vi "Find Xbee.vi"(8 "error out":errorcluster, 11 "Aircraft COM Port":refnum<visa-resource-name>) -> (0 "error out 2":errorcluster, 2 "Xbee Found":bool, 3 "Aircraft COM Port 2":refnum<visa-resource-name>)   [LabVIEW 2014]
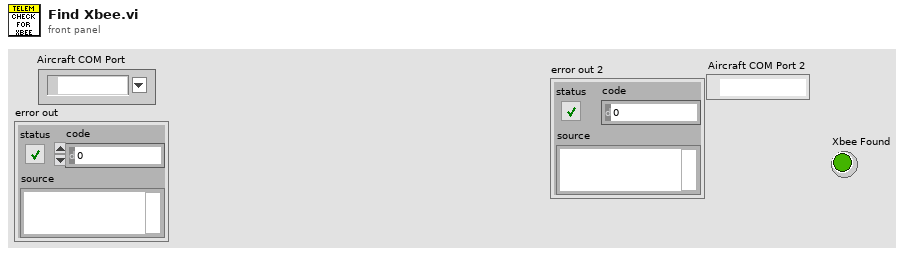
[diagram p1: front panel]
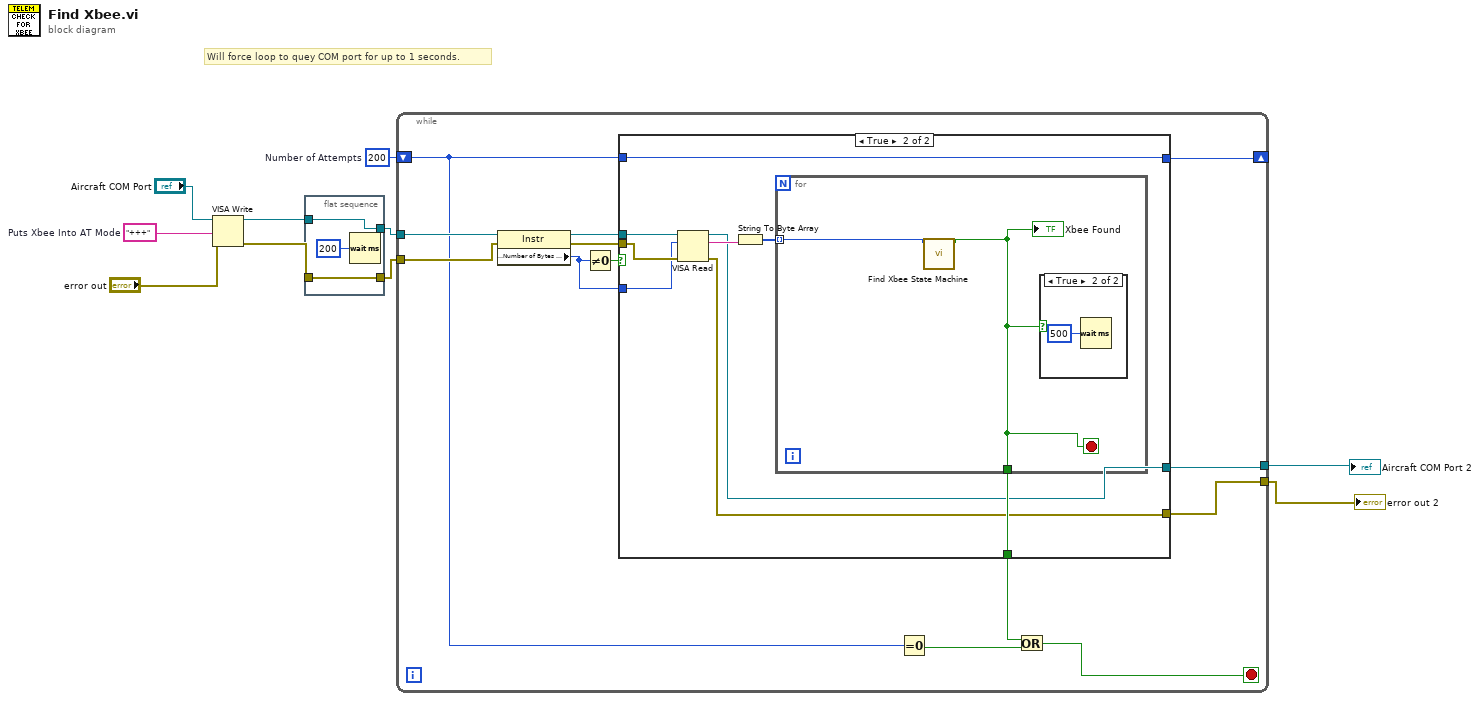
[diagram p0: block diagram]
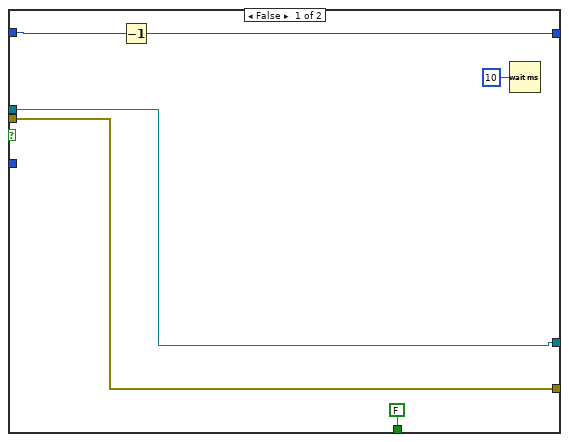
[diagram p2: hidden frame]
diagram:
  w9 = "+++"  # Puts Xbee Into AT Mode
  w10 = 200  # Number of Attempts
  # "Will force loop to quey COM port for up to 1 seconds."
  n1 = VISA Write(VISA resource name="Aircraft COM Port", write buffer=w9, error in (no error)="error out") -> (VISA resource name out=w8:refnum<visa-resource-name>, error out=w6:errorcluster)  [unwired: 1 out]
  n2 = flat-sequence {
    tunnel: w8 -> [w12]
    tunnel: [w12] -> w7
    tunnel: w6 -> [w11]
    tunnel: [w11] -> w5
    frame #0 {
      n3 = Wait (ms)(milliseconds to wait=u32 200) -> ()  [unwired: 1 out]
    }
  }
  n4 = while {
    tunnel: w7 -> [w26]
    tunnel: w5 -> [w25]
    tunnel: [w20] -> w1
    tunnel: [w19] -> w2
    shift-right: [w18] -> _
    shift-left: w10 -> [w14]
    stop <- w15 stop-if-true
    n5 = property class="Instr"(reference=w26, error in=w25) -> (reference out=w23:refnum<visa-resource-name>, error out=w22:errorcluster, "Serial Settings:Number of Bytes at Serial Port"=w21:u32)
    n6 = Not Equal To 0?(x=w21) -> (x != 0?=w24:bool)
    n7 = case shown="True" w24 {
      tunnel: w23 -> [w30 w41]
      tunnel: w22 -> [w31 w40]
      tunnel: w21 -> [_ w39]
      tunnel: [FALSE ("Message Complete") w36] -> w17
      tunnel: [w31 w35] -> w20
      tunnel: [w30 w34] -> w19
      tunnel: w14 -> [w28 w33]
      tunnel: [w27 w33] -> w18
      frame False {
        n8 = Decrement(x=w28) -> (x-1=w27:i32)
        n9 = Wait (ms)(milliseconds to wait=u32 10) -> ()  [unwired: 1 out]
      }
      frame True {
        n10 = VISA Read(VISA resource name=w41, byte count=w39, error in (no error)=w40) -> (VISA resource name out=w34:refnum<visa-resource-name>, read buffer=w38:string, error out=w35:errorcluster)  [unwired: 1 out]
        n11 = String To Byte Array(string=w38) -> (unsigned byte array=w37:u8[])
        n12 = for {
          tunnel: w37 -> [w43] mode=indexing
          tunnel: [w42] -> w36
          stop <- w42 stop-if-true
          n13 = call "Find Xbee State Machine.vi"("Incoming Bytes"=w43) -> ("Xbee Found"=w42:bool)  [unwired: 10 in]
          "Xbee Found" <- w42
          n14 = case shown="True" w42 {
            frame False {
            }
            frame True {
              n15 = Wait (ms)(milliseconds to wait=u32 500) -> ()  [unwired: 1 out]
            }
          }
        }
      }
    }
    n16 = Equal To 0?(x=w14) -> (x = 0?=w16:bool)
    n17 = Or(x=w17, y=w16) -> (x .or. y?=w15:bool)
  }
  "error out 2" <- w1
  "Aircraft COM Port 2" <- w2
